vi "Windows.Exit.vi"(7 "Exit Action":T1=enum."Shut Down PC") -> (0 "error out":errorcluster)   [LabVIEW 2016]
doc: "This VI allows you to exit windows in various ways.\nexit windows function\n0: Log off\n1: Shut Down\n2: Exit Windows and reboot the computer"
uses:
  Windows.ExitAction.ctl
  user32.dll
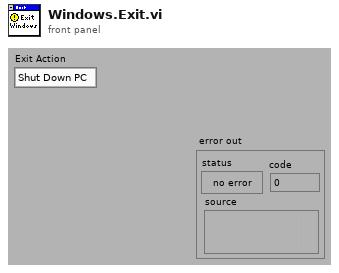
[diagram p1: front panel]
types:
  T1 = typedef "Windows.ExitAction.ctl" = enum16{"Log off from PC", "Shut Down PC", "Reboot PC", "Close Program"}
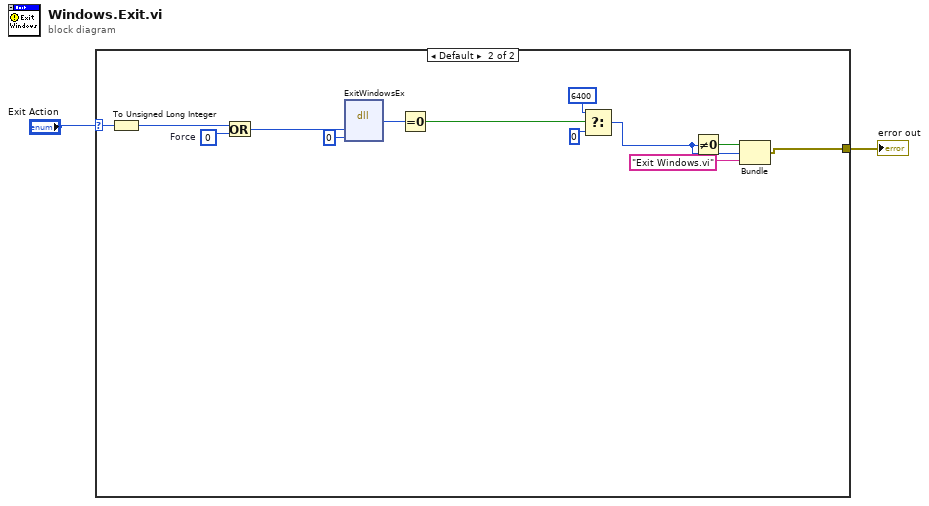
[diagram p0: block diagram]
diagram:
  n1 = case shown="Default" "Exit Action" {
    selector: "Exit Action" -> [_ w8]
    tunnel: [_ w6] -> w2
    frame "Close Program" {
    }
    frame Default {
      w10 = u32 0  # Force
      n2 = To Unsigned Long Integer(number=w8) -> (unsigned 32bit integer=w3:u32)
      n3 = Or(x=w3, y=w10) -> (x .or. y?=w9:u32)
      n4 = dll-call lib="User32.dll" fn="ExitWindowsEx" label="ExitWindows"("returnCode"=w9, "reserved (set to zero)"=u32 0) -> (w11:i32)  [unwired: 5 in, 2 out]
      n5 = Equal To 0?(x=w11) -> (x = 0?=w7:bool)
      n6 = Select(t=6400, s=w7, f=0) -> (s? t:f=w14:i32)
      n7 = Not Equal To 0?(x=w14) -> (x != 0?=w15:bool)
      n8 = Bundle(w15, w14, "Exit Windows.vi") -> (w6:errorcluster)  [unwired: 1 out]
    }
  }
  "error out" <- w2
